vi "P2Y2.vi"() -> ()   [LabVIEW 2020]
panel:
  in  "stop":bool
  out "Waveform Graph":cluster{i32, i32, dbl[]}[](graph)
  in  "cos amp":dbl
  in  "sin amp":dbl
  in  "cos sagedus":i32
  in  "sin sagedus":u32
  in  "Puntkide arv":i32
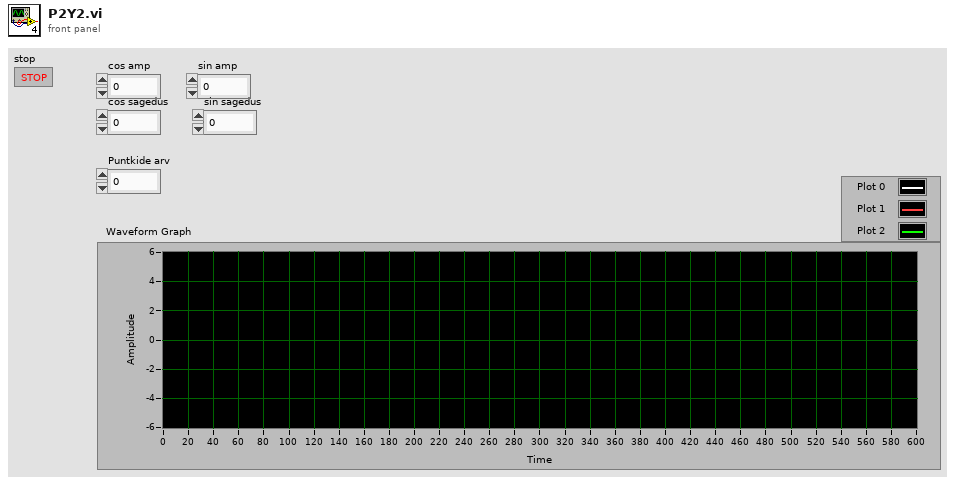
[diagram p1: front panel]
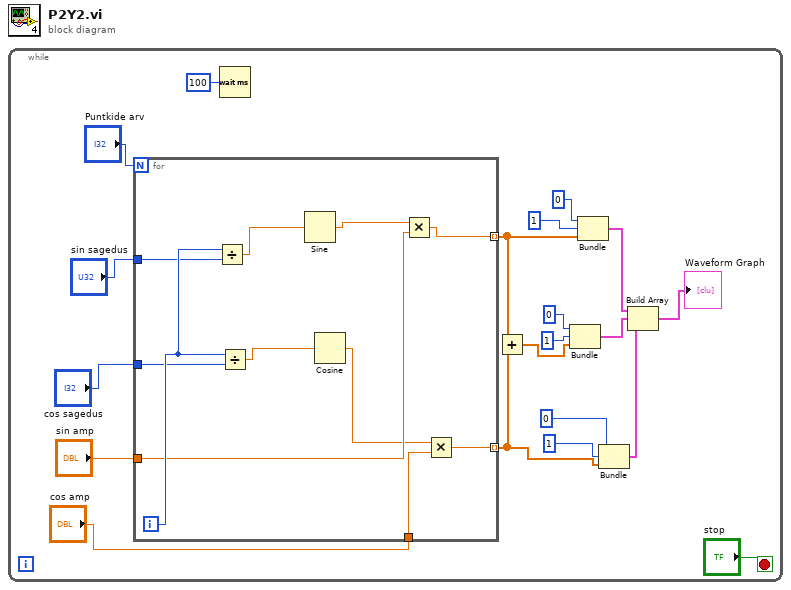
[diagram p0: block diagram]
diagram:
  n1 = while {
    stop <- "stop" stop-if-true
    n2 = for {
      N: "Puntkide arv" -> [_]
      tunnel: "sin sagedus" -> [w30]
      tunnel: "cos sagedus" -> [w29]
      tunnel: "sin amp" -> [w26]
      tunnel: "cos amp" -> [w25]
      tunnel: [w22] -> w8 mode=indexing
      tunnel: [w21] -> w10 mode=indexing
      i -> [w31]
      n3 = Divide(x=w31, y=w30) -> (x/y=w27:dbl)
      n4 = Divide(x=w31, y=w29) -> (x/y=w28:dbl)
      n5 = Sine(x=w27) -> (sin(x)=w24:dbl)
      n6 = Cosine(x=w28) -> (cos(x)=w23:dbl)
      n7 = Multiply(x=w24, y=w26) -> (x*y=w21:dbl)
      n8 = Multiply(x=w23, y=w25) -> (x*y=w22:dbl)
    }
    n9 = Wait (ms)(milliseconds to wait=u32 100) -> ()  [unwired: 1 out]
    n10 = Add(x=w10, y=w8) -> (x+y=w9:dbl[])
    n11 = Bundle(0, 1, w9) -> (w4:cluster{i32, i32, dbl[]})  [unwired: 1 in]
    n12 = Bundle(0, 1, w10) -> (w5:cluster{i32, i32, dbl[]})  [unwired: 1 in]
    n13 = Bundle(0, 1, w8) -> (w3:cluster{i32, i32, dbl[]})  [unwired: 1 in]
    n14 = Build Array(w5, w4, w3) -> (→"Waveform Graph":cluster{i32, i32, dbl[]}[])
  }
